vi "OutputChannelSignalGet.vi"(0 "SR865 in":T3, 2 "OutputChannel":T2 caption="Output channel" items=["Channel 1", "Channel 2"], 5 "error in":errorcluster) -> (14 "SR865 out":T3, 16 "OutputChannelSignal":T1 caption="Output channel signal" items=["X (ch1) / Y (ch2)", "R (ch1) / Q (ch2)"], 19 "error out":errorcluster)   [LabVIEW 2017]
uses:
  SR865.ctl
  OutputChannel.ctl
  OutputChannelSignal.ctl
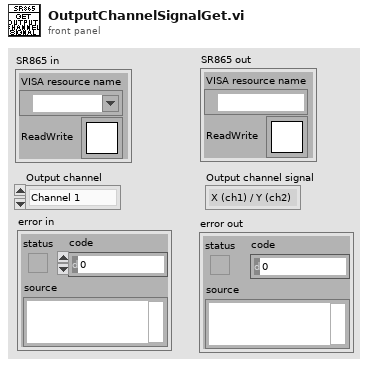
[diagram p1: front panel]
types:
  T1 = typedef "OutputChannelSignal.ctl" = u16
  T2 = typedef "OutputChannel.ctl" = u16
  T3 = typedef "SR865.ctl" = cluster{"VISA resource name":refnum<visa-resource-name>, "ReadWrite":T4}
  T4 = typedef "Semaphore RefNum" = refnum<k1>
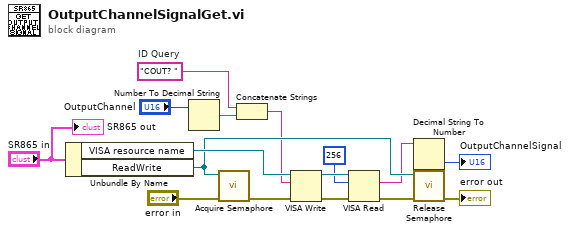
[diagram p0: block diagram]
diagram:
  w4 = "COUT? "  # ID Query
  n1 = Unbundle By Name("SR865 in") -> ("VISA resource name"=w12:refnum<visa-resource-name>, "ReadWrite"=w7:T4)
  n2 = Number To Decimal String(number="OutputChannel") -> (decimal integer string=w2:string)  [unwired: 1 in]
  n3 = call <vilib>:"Acquire Semaphore.vi"("error in (no error)"="error in", "semaphore"=w7) -> ("error out"=w11:errorcluster)  [unwired: 3 in, 2 out]
  n4 = Concatenate Strings(w4, w2) -> (w1:string)
  n5 = VISA Write(VISA resource name=w12, write buffer=w1, error in (no error)=w11) -> (VISA resource name out=w15:refnum<visa-resource-name>, error out=w14:errorcluster)  [unwired: 1 out]
  n6 = VISA Read(VISA resource name=w15, byte count=u32 256, error in (no error)=w14) -> (read buffer=w6:string, error out=w9:errorcluster)  [unwired: 2 out]
  n7 = Decimal String To Number(string=w6) -> (number=→"OutputChannelSignal":i32)  [unwired: 2 in, 1 out]
  n8 = call <vilib>:"Release Semaphore.vi"("error in (no error)"=w9, "semaphore"=w7) -> ("error out"=→"error out":errorcluster)  [unwired: 4 in, 1 out]
  "SR865 out" <- "SR865 in"
